vi "DiagDeviceControl.vi"(10 "Enum":T1, 11 "Device":string) -> (1 "concatenated string":string, 2 "IP Addresses":string[](array[string]), 3 "Ports":string[](array[string]))   [LabVIEW 2020]
uses:
  Controls/DeviceControl_Typdef.ctl
  Shared/MySQL/Preset Query Enum.ctl
panel:
  out "element":string
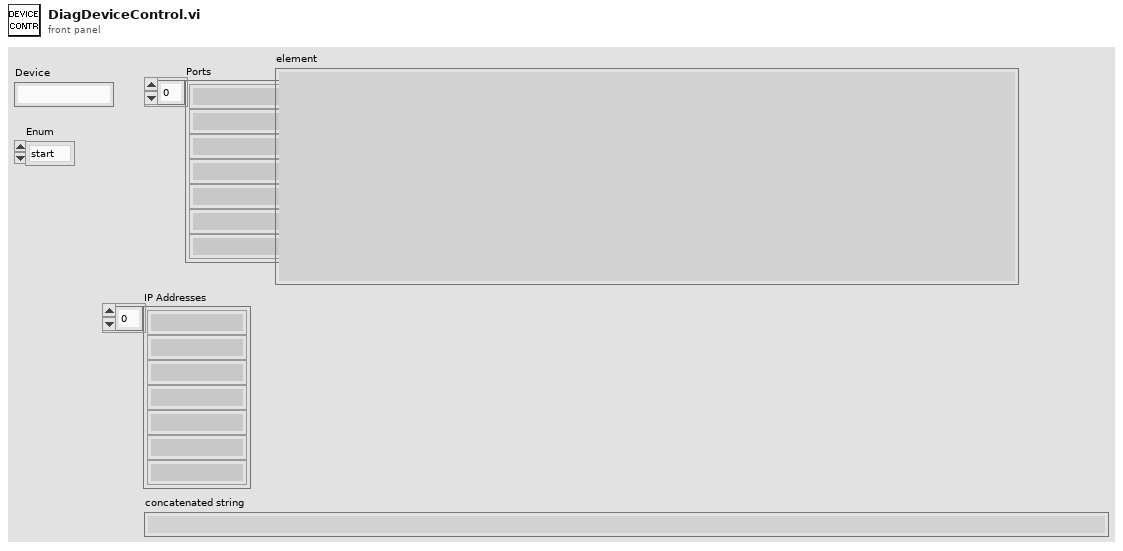
[diagram p1: front panel]
types:
  T1 = typedef "DeviceControl_Typdef.ctl" = enum16{"start", "stop", "kill", "PC rdp", "PC start", "PC shutdown", "PC restart", "GUI start"}
  T2 = typedef "Preset Query Enum.ctl" = enum16{"Get Locations", "Get all IPs and MACs", "Get classes", "Get expt variables to set at scanstart for particular device", "Get expt devices and variables with start values", "Get expt devices and variables (with data to get)", "Get expt devices with data to get", "Get Expt devices and GUIs", "Get all devices basic properties", "Get Virtual Devices Core Info", "Get Expt names", "Get experiment basic properties", "Get experiment alarm variables", "Get MC Ports", "Get device network comm port", "Get devicetype lvclass path", "Get basic device properties", "Get Init Order", "Get all setable variables of a device", "Get device variable aliases", "Get force values of all settable variables", "Get all variables of a devicetype", "Get all variables of a device", "Get plotter details", "Get Saved Scans", "Get Scan Info", "GetGeneralGUIs", "Get expt for plotter", "Get plotter IDs from expt", "Get all devices", "Get all Virtual Devices", "Get all aliases", "Get variable and device info for Virtual Device", "GetItemLocatorIP", "Get IPs for GUIs", "Get DeviceType from Device", "GetLocalPortRange", "GetDevicePresetVariables", "Get Device Configuration", "GetAllPresetNames", "GetAllConfigurationNames", "GetPresetDeviceNames", "GetDeviceAliases", "GetDevicesOfClass"}
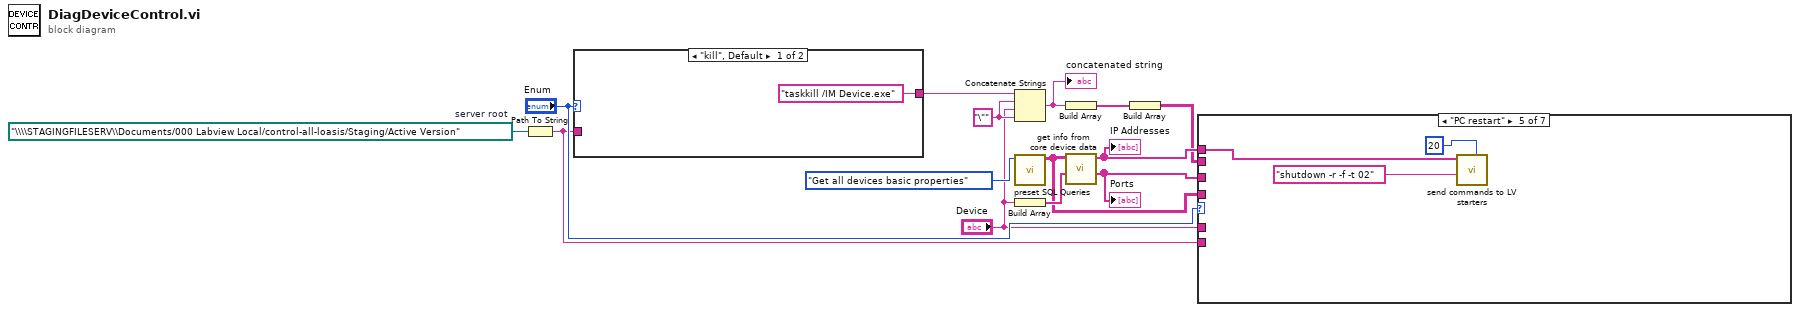
[diagram p0: block diagram]
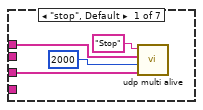
[diagram p2: hidden frame]
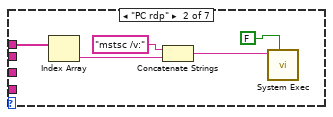
[diagram p3: hidden frame]
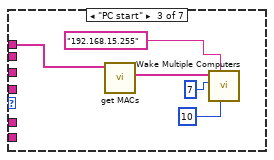
[diagram p4: hidden frame]
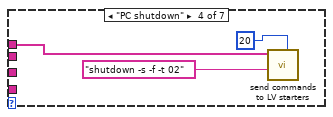
[diagram p5: hidden frame]
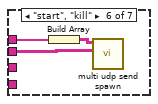
[diagram p6: hidden frame]
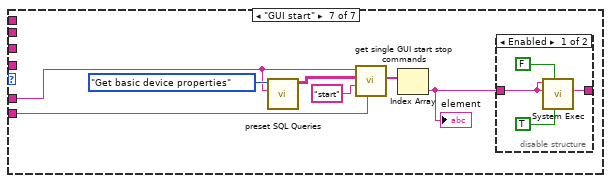
[diagram p7: hidden frame]
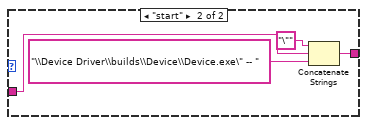
[diagram p9: hidden frame]
diagram:
  w7 = "\"" ("string")
  w1 = path "\\\\STAGINGFILESERV\\Documents/000 Labview Local/control-all-loasis/Staging/Active Version"  # server root
  n1 = Path To String(path=w1) -> (string=w3:string)
  n2 = case shown="\"kill\", Default" "Enum" {
    tunnel: ["taskkill /IM Device.exe" ("Class") w19] -> w8
    tunnel: w3 -> [_ w16]
    frame "kill", Default {
    }
    frame "start" {
      n3 = Concatenate Strings("\"" ("string"), w16, "\\Device Driver\\builds\\Device\\Device.exe\" -- " ("Class")) -> (w19:string)
    }
  }
  n4 = Concatenate Strings(w8, w7, "Device", w7) -> (w9:string)
  "concatenated string" <- w9
  n5 = call "preset SQL Queries.vi"("Preset Query"=Preset_Query_Enum."Get all devices basic properties") -> ("data"=w2:string[][])  [unwired: 8 in, 2 out]
  n6 = Build Array("Device") -> (w6:string[])
  n7 = Build Array(w9) -> (w10:string[])
  n8 = call "get info from core device data.vi"("devices to get data from"=w6, "All Devices Core Info"=w2) -> ("Ports"=w13:string[], "IP Addresses"=w12:string[])  [unwired: 1 in, 3 out]
  "IP Addresses" <- w12
  "Ports" <- w13
  n9 = Build Array(w10) -> (w11:string[][])
  n10 = case shown="\"PC restart\"" "Enum" {
    tunnel: w11 -> [_ _ _ _ _ w42 _]
    tunnel: w12 -> [w21 w24 w29 w34 w37 w41 _]
    tunnel: w13 -> [w20 _ _ _ _ _ _]
    tunnel: "Device" -> [_ _ _ _ _ _ w46]
    tunnel: w3 -> [_ _ _ _ _ _ w49]
    tunnel: w2 -> [_ _ _ _ _ _ _]
    frame "stop", Default {
      n11 = call "udp multi alive.vi"("command"="Stop", "IPs"=w21, "timeout ms (25000)"=2000, "remote Ports"=w20) -> ()  [unwired: 2 in, 2 out]
    }
    frame "PC rdp" {
      n12 = Index Array(array=w24) -> (element=w26:string)  [unwired: 1 in]
      n13 = Concatenate Strings("mstsc /v:" ("IP"), w26) -> (w28:string)
      n14 = call <vilib>:"System Exec.vi"("wait until completion? (T)"=FALSE, "command line"=w28) -> ()  [unwired: 4 in, 6 out]
    }
    frame "PC start" {
      n15 = call "get MACs.vi"("IP Addresses to..."=w29) -> ("MACs Hex"=w32:string[])  [unwired: 9 in, 1 out]
      n16 = call "Wake Multiple Computers.vi"("wait in between [ms]"=u32 10, "Broadcast IP-address"="192.168.15.255", "local port"=u16 7, "MAC Addresses to Start"=w32) -> ()  [unwired: 7 in, 1 out]
    }
    frame "PC shutdown" {
      n17 = call "send commands to LV starters.vi"("IP Addresses"=w34, "Message"="shutdown -s -f -t 02", "time between commands (ms)"=u32 20) -> ()  [unwired: 5 in, 2 out]
    }
    frame "PC restart" {
      n18 = call "send commands to LV starters.vi"("IP Addresses"=w37, "Message"="shutdown -r -f -t 02", "time between commands (ms)"=u32 20) -> ()  [unwired: 5 in, 2 out]
    }
    frame "start", "kill" {
      n19 = Build Array(w41) -> (w40:string[][])
      n20 = call "multi udp send spawn.vi"("IP array"=w40, "Message array"=w42) -> ()  [unwired: 6 in, 1 out]
    }
    frame "GUI start" {
      n21 = call "preset SQL Queries.vi"("Device/Devicetype name\n/Plotter.id/ScanName#"=w46, "Preset Query"=Preset_Query_Enum."Get basic device properties") -> ("data"=w45:string[][])  [unwired: 7 in, 2 out]
      n22 = call "get single GUI start stop commands.vi"("Software root"=w49, "Argument (start stop kill)"="start", "active device basic properties"=w45, "active device"=w46) -> ("GUI start/stop commands"=w44:string[])  [unwired: 7 in]
      n23 = Index Array(array=w44) -> (element=w43:string)  [unwired: 1 in]
      "element" <- w43
      n24 = disable-structure shown="Enabled" {
        disable-tunnel: w43 -> [w51 _]
        disable-tunnel: [w52 _] -> _
        frame Enabled {
          n25 = call <vilib>:"System Exec.vi"("run minimized? (F)"=TRUE, "wait until completion? (T)"=FALSE, "standard input"=w51, "command line"=w51) -> ("standard error"=w52:string)  [unwired: 2 in, 5 out]
        }
        frame Disabled {
        }
      }
    }
  }
